vi "TProfile_selector_GeoCal_RangeWalk.vi"() -> (1 "TestType":string="Geocal", 3 "Path":path=path "C:/luminartech/ManufacturingTools/TS_Automation/Data/ORD/TestProfile_OP80_Reflectance_Rev2p3.csv")   [LabVIEW 2018]
panel:
  in  "Start Button 3":bool
  in  "Start Button 2":bool
  in  "Start Button":bool
  # "GeoCal & RangeWalk Test station"
  # "Test Profile Selector"
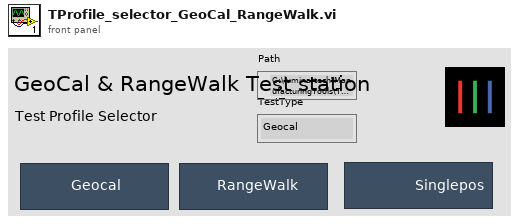
[diagram p1: front panel]
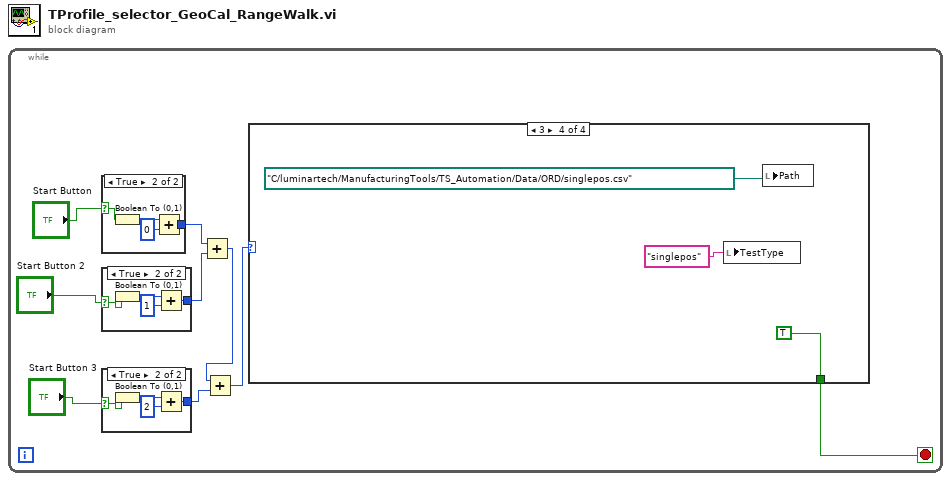
[diagram p0: block diagram]
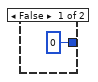
[diagram p2: hidden frame]
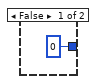
[diagram p3: hidden frame]
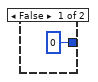
[diagram p4: hidden frame]
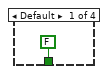
[diagram p5: hidden frame]
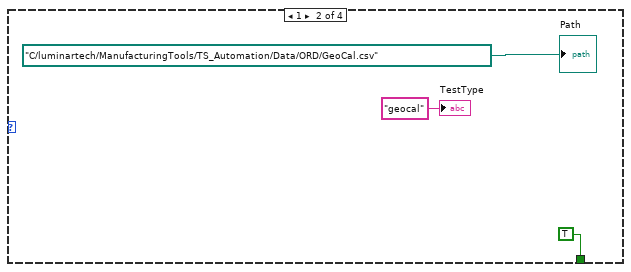
[diagram p6: hidden frame]
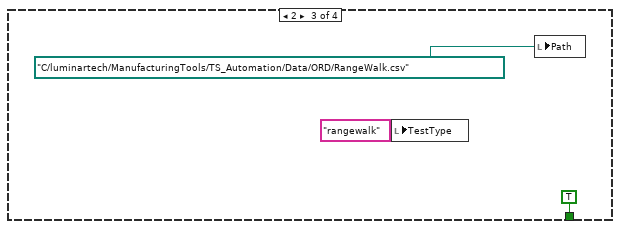
[diagram p7: hidden frame]
diagram:
  n1 = while {
    stop <- w7 stop-if-true
    n2 = case shown="True" "Start Button" {
      selector: "Start Button" -> [_ w16]
      tunnel: [i16 0 w17] -> w9
      frame False {
      }
      frame True {
        n3 = Boolean To (0,1)(Boolean=w16) -> (0, 1=w19:i16)
        n4 = Add(x=w19, y=i16 0) -> (x+y=w17:i16)
      }
    }
    n5 = case shown="True" "Start Button 2" {
      selector: "Start Button 2" -> [_ w21]
      tunnel: [i16 0 w22] -> w8
      frame False {
      }
      frame True {
        n6 = Boolean To (0,1)(Boolean=w21) -> (0, 1=w24:i16)
        n7 = Add(x=w24, y=i16 1) -> (x+y=w22:i16)
      }
    }
    n8 = case shown="True" "Start Button 3" {
      selector: "Start Button 3" -> [_ w11]
      tunnel: [i16 0 w12] -> w3
      frame False {
      }
      frame True {
        n9 = Boolean To (0,1)(Boolean=w11) -> (0, 1=w14:i16)
        n10 = Add(x=w14, y=i16 2) -> (x+y=w12:i16)
      }
    }
    n11 = Add(x=w9, y=w8) -> (x+y=w2:i16)
    n12 = Add(x=w2, y=w3) -> (x+y=w1:i16)
    n13 = case shown="3" w1 {
      tunnel: [FALSE TRUE TRUE TRUE] -> w7
      frame Default {
      }
      frame 1 {
        "Path" <- path "C:/luminartech/ManufacturingTools/TS_Automation/Data/ORD/GeoCal.csv"
        "TestType" <- "geocal"
      }
      frame 2 {
        n14 = local write "TestType"("rangewalk" ("TestType")) -> ()
        n15 = local write "Path"(path "C:/luminartech/ManufacturingTools/TS_Automation/Data/ORD/RangeWalk.csv") -> ()
      }
      frame 3 {
        n16 = local write "TestType"("singlepos" ("TestType")) -> ()
        n17 = local write "Path"(path "C:/luminartech/ManufacturingTools/TS_Automation/Data/ORD/singlepos.csv") -> ()
      }
    }
  }
